vi "FunctionGenerator.vi"() -> ()   [LabVIEW 2017]
uses:
  waveformctrlFG.ctl
  FunctionGeneratorControls.ctl
  <vilib>/DAQmx/write.llb/DAQmx Write (Analog 1D DBL 1Chan NSamp).vi
  <vilib>/DAQmx/create/channels.llb/DAQmx Create Channel (AO-Voltage-Basic).vi
  <vilib>/DAQmx/configure/timing.llb/DAQmx Timing (Sample Clock).vi
  <vilib>/DAQmx/miscellaneous.llb/DAQmx Fill In Error Info.vi
  <resource>/objmgr/daqmx.rc
panel:
  in  "physical channels":tag="Dev8/ao0"
  in  "Frequency":dbl=1000.0 min=1.0 max=100000.0 step=1.0
  in  "Duty Cycle":dbl(knob)=0.5 min=0.1 max=0.99 step=0.1 scale=0.1..0.99
  in  "DC Offset":dbl(knob) min=-10.0 max=10.0 step=1.0 scale=-10.0..10.0
  in  "Amplitude":dbl(knob)=9.99 min=1.0 max=9.99 scale=1.0..10.0
  in  "Waveform":T1 items=["Sine", "Triangle", "Sawtooth", "Square", "TTL"]
  in  "stop":bool
  out "Waveform Graph":dbl[](graph)=[0.0, 0.07846046987822623, 0.15691609994508854, 0.23536205068776545, 0.31379348319050165, 0.39220555943309543, 0.4705934425893302, 0.5489522973253331, 0.6272772900978406, 0.7055635894523551, 0.783806366321171, 0.8620007943212546, 0.9401420500519582, 1.0182253133925498, 1.0962457677995423, 1.1741986006037983, 1.2520790033073996, 1.329882171880258, 1.4076033070564509, 1.4852376146302608, 1.5627803057519065, 1.6402265972229408, 1.7175717117913014, 1.7948108784459935, 1.8719393327113891, 1.9489523169411216, 2.02584508061156, 2.102612880614844, 2.1792509815514602, 2.2557546560223463, 2.332119184920495, 2.4083398577220563, 2.4844119727768996, 2.5603308375986367, 2.6360917691540755, 2.711690094152092, 2.7871211493319006, 2.8623802817507054, 2.937462849070717, 3.0123642198455123, 3.0870797738057245, 3.1616049021440453, 3.2359350077995126, 3.3100655057410844, 3.3839918232504616, 3.4577094002041555, 3.5312136893547788, 3.6045001566115418, 3.677564281319933, 3.750401556540578, 3.8230074893272477, 3.8953776010040007, 3.9675074274414586, 4.0393925193321625, 4.111028442465037, 4.182410777998907, 4.253535122735077, 4.324397089388936, 4.394992306860592, 4.4653164205045, 4.535365092398073, 4.60513400160927, 4.6746188444631285, 4.74381533480724, 4.812719204276136, 4.88132620255458, 4.949632097639752, 5.017632676102291, 5.085323743346209, 5.152701123867625, 5.219760661512328, 5.286498219732165, 5.352909681840177, 5.418990951264557, 5.484737951801336, 5.550146627865826, 5.615212944742785, 5.679932888835297, 5.744302467912353, 5.808317711355108, 5.871974670401807, 5.935269418391366, 5.9981980510055815, 6.060756686509977, 6.122941465993235, 6.1847485536052424, 6.246174136793695, 6.307214426539284, 6.367865657589411, 6.428124088690452, 6.487986002818536, 6.547447707408821, 6.606505534583282, 6.665155841376952, 6.723395009962635, 6.781219447874088, 6.8386255882276, 6.895609889942028, 6.952168837957221, 7.008298943450849, 7.06399674405361, 7.119258804062802, 7.174081714654257, 7.2284620940926105, 7.2823965879399015, 7.335881869262499, 7.388914638836311, 7.441491625350304, 7.493609585608292, 7.545265304728985, 7.596455596344311, 7.64717730279595, 7.697427295330135, 7.7472024742906225, 7.796499769309913, 7.845316139498642, 7.893648573633147, 7.9414940903412266, 7.988849738286035, 8.035712596348144, 8.082079773805726, 8.127948410512863, 8.173315677075985, 8.21817877502839, 8.262534937002872, 8.306381426902426, 8.34971554006902, 8.39253460345043, 8.43483597576513, 8.476617047665222, 8.51787524189738, 8.558608013461848, 8.598812849769397, 8.63848727079635, 8.67762882923753, 8.716235110657243, 8.7543037336382, 8.791832349928407, 8.828818644586049, 8.86526033612224, 8.901155176641794, 8.936500951981872, 8.97129548184855, 9.005536619951334, 9.039222254135536, 9.072350306512561, 9.104918733588098, 9.13692552638815, 9.168368710582971, 9.199246346608852, 9.229556529787756, 9.259297390444807, 9.288467094023632, 9.317063841199511, 9.345085867990374, 9.372531445865617, 9.399398881852713, 9.425686518641655, 9.451392734687177, 9.47651594430879, 9.501054597788585, 9.525007181466822, 9.548372217835318, 9.571148265628569, 9.593333919912661, 9.614927812171937, 9.635928610393403, 9.656335019148905, 9.676145779675025, 9.69535966995074, 9.71397550477279, 9.731992135828795, 9.749408451768087, 9.76622337827026, 9.78243587811144, 9.798044951228272, 9.8130496347796, 9.827449003205864, 9.841242168286191, 9.85442827919319, 9.867006522545427, 9.878976122457601, 9.89033634058841, 9.901086476186089, 9.911225866131634, 9.920753884979714, 9.929669944997245, 9.937973496199648, 9.945664026384769, 9.952741061164483, 9.959204163993949, 9.96505293619854, 9.970287016998434, 9.974906083530874, 9.97890985087008, 9.982298072044822, 9.985070538053659, 9.987227077877826, 9.988767558491789, 9.98969188487145, 9.99, 9.98969188487145, 9.988767558491789, 9.987227077877826, 9.985070538053659, 9.982298072044822, 9.97890985087008, 9.974906083530874, 9.970287016998434, 9.965052936198537, 9.959204163993949, 9.952741061164483, 9.945664026384769, 9.937973496199648, 9.929669944997245, 9.920753884979714, 9.911225866131634, 9.901086476186087, 9.89033634058841, 9.878976122457601, 9.867006522545426, 9.85442827919319, 9.841242168286191, 9.827449003205864, 9.813049634779599, 9.798044951228272, 9.78243587811144, 9.76622337827026, 9.749408451768087, 9.731992135828795, 9.713975504772788, 9.69535966995074, 9.676145779675025, 9.656335019148903, 9.635928610393403, 9.614927812171937, 9.593333919912661, 9.571148265628569, 9.548372217835318, 9.525007181466822, 9.501054597788585, 9.47651594430879, 9.451392734687177, 9.425686518641655, 9.399398881852713, 9.372531445865615, 9.345085867990374, 9.317063841199511, 9.288467094023632, 9.259297390444805, 9.229556529787756, 9.199246346608852, 9.168368710582971, 9.136925526388149, 9.104918733588098, 9.072350306512561, 9.039222254135534, 9.005536619951334, 8.97129548184855, 8.936500951981872, 8.901155176641796, 8.865260336122239, 8.828818644586045, 8.791832349928407, 8.754303733638196, 8.716235110657243, 8.67762882923753, 8.63848727079635, 8.598812849769397, 8.558608013461846, 8.517875241897382, 8.47661704766522, 8.43483597576513, 8.392534603450429, 8.349715540069019, 8.306381426902426, 8.262534937002872, 8.21817877502839, 8.173315677075983, 8.127948410512863, 8.082079773805726, 8.035712596348143, 7.988849738286033, 7.941494090341224, 7.893648573633146, 7.8453161394986415, 7.796499769309913, 7.7472024742906225, 7.697427295330135, 7.64717730279595, 7.596455596344309, 7.545265304728983, 7.493609585608289, 7.441491625350303, 7.38891463883631, 7.335881869262498, 7.282396587939901, 7.228462094092609, 7.174081714654257, 7.119258804062802, 7.06399674405361, 7.008298943450846, 6.952168837957219, 6.895609889942025, 6.838625588227599, 6.781219447874087, 6.723395009962635, 6.665155841376951, 6.606505534583282, 6.547447707408821, 6.487986002818536, 6.428124088690449, 6.367865657589409, 6.307214426539281, 6.246174136793694, 6.184748553605241, 6.122941465993234, 6.0607566865099765, 5.9981980510055815, 5.935269418391366, 5.871974670401808, 5.808317711355105, 5.744302467912351, 5.679932888835295, 5.615212944742783, 5.550146627865826, 5.4847379518013355, 5.418990951264556, 5.352909681840177, 5.286498219732165, 5.219760661512327, 5.1527011238676215, 5.0853237433462075, 5.01763267610229, 4.94963209763975, 4.881326202554579, 4.812719204276135, 4.74381533480724, 4.6746188444631285, 4.60513400160927, 4.535365092398069, 4.4653164205044975, 4.3949923068605905, 4.324397089388934, 4.253535122735074, 4.182410777998905, 4.111028442465036, 4.0393925193321625, 3.9675074274414586, 3.8953776010040015, 3.8230074893272437, 3.750401556540575, 3.6775642813199307, 3.60450015661154, 3.5312136893547774, 3.4577094002041537, 3.38399182325046, 3.310065505741084, 3.235935007799513, 3.161604902144046, 3.087079773805722, 3.012364219845509, 2.937462849070714, 2.862380281750703, 2.787121149331899, 2.711690094152091, 2.6360917691540746, 2.5603308375986362, 2.4844119727768996, 2.408339857722057, 2.332119184920492, 2.255754656022343, 2.1792509815514576, 2.1026128806148416, 2.025845080611558, 1.9489523169411205, 1.8719393327113885, 1.7948108784459935, 1.7175717117913016, 1.6402265972229415, 1.5627803057519032, 1.485237614630258, 1.4076033070564484, 1.3298821718802563, 1.2520790033073979, 1.1741986006037972, 1.0962457677995416, 1.0182253133925498, 0.9401420500519584, 0.8620007943212509, 0.7838063663211678, 0.7055635894523523, 0.6272772900978383, 0.5489522973253311, 0.4705934425893287, 0.3922055594330944, 0.3137934831905011, 0.23536205068776533, 0.1569160999450889, 0.07846046987822257, -3.21302905405392e-15, -0.07846046987822898, -0.15691609994509087, -0.2353620506877673, -0.3137934831905031, -0.3922055594330964, -0.4705934425893307, -0.5489522973253331, -0.6272772900978404, -0.7055635894523589, -0.7838063663211742, -0.8620007943212573, -0.9401420500519604, -1.0182253133925516, -1.0962457677995436, -1.174198600603799, -1.2520790033073999, -1.329882171880258, -1.4076033070564502, -1.4852376146302644, -1.5627803057519094, -1.6402265972229435, -1.7175717117913036, -1.7948108784459953, -1.8719393327113905, -1.9489523169411223, -2.02584508061156, -2.102612880614844, -2.17925098155146, -2.2557546560223494, -2.332119184920498, -2.408339857722059, -2.484411972776902, -2.5603308375986384, -2.636091769154077, -2.7116900941520923, -2.7871211493319006, -2.8623802817507054, -2.937462849070716, -3.012364219845515, -3.087079773805728, -3.1616049021440475, -3.235935007799515, -3.310065505741086, -3.383991823250462, -3.457709400204156, -3.5312136893547788, -3.6045001566115418, -3.6775642813199365, -3.7504015565405813, -3.82300748932725, -3.8953776010040038, -3.9675074274414603, -4.039392519332164, -4.111028442465038, -4.182410777998907, -4.253535122735076, -4.324397089388935, -4.394992306860596, -4.465316420504503, -4.5353650923980755, -4.605134001609271, -4.67461884446313, -4.743815334807242, -4.812719204276137, -4.881326202554581, -4.949632097639752, -5.017632676102291, -5.085323743346213, -5.152701123867627, -5.219760661512332, -5.286498219732166, -5.352909681840178, -5.418990951264558, -5.484737951801336, -5.550146627865827, -5.615212944742785, -5.679932888835297, -5.744302467912356, -5.8083177113551105, -5.871974670401809, -5.935269418391367, -5.998198051005583, -6.060756686509978, -6.122941465993236, -6.1847485536052424, -6.246174136793695, -6.307214426539284, -6.367865657589413, -6.4281240886904545, -6.487986002818537, -6.547447707408824, -6.606505534583284, -6.665155841376952, -6.723395009962637, -6.781219447874088, -6.8386255882276, -6.895609889942028, -6.952168837957222, -7.008298943450851, -7.063996744053611, -7.119258804062804, -7.174081714654258, -7.2284620940926105, -7.2823965879399015, -7.335881869262499, -7.388914638836311, -7.441491625350304, -7.493609585608294, -7.5452653047289875, -7.5964555963443114, -7.647177302795949, -7.697427295330136, -7.747202474290626, -7.796499769309915, -7.845316139498646, -7.893648573633147, -7.941494090341228, -7.988849738286034, -8.035712596348146, -8.082079773805724, -8.127948410512865, -8.173315677075987, -8.21817877502839, -8.262534937002876, -8.306381426902426, -8.349715540069022, -8.39253460345043, -8.434835975765132, -8.47661704766522, -8.517875241897384, -8.558608013461845, -8.598812849769399, -8.638487270796352, -8.67762882923753, -8.716235110657246, -8.754303733638197, -8.791832349928411, -8.828818644586047, -8.86526033612224, -8.901155176641794, -8.936500951981872, -8.971295481848554, -9.005536619951336, -9.039222254135538, -9.072350306512563, -9.1049187335881, -9.136925526388149, -9.168368710582973, -9.199246346608852, -9.229556529787756, -9.259297390444805, -9.288467094023632, -9.317063841199513, -9.345085867990376, -9.372531445865619, -9.399398881852713, -9.425686518641655, -9.451392734687177, -9.476515944308792, -9.501054597788585, -9.525007181466822, -9.54837221783532, -9.571148265628569, -9.593333919912663, -9.614927812171937, -9.635928610393405, -9.656335019148903, -9.676145779675025, -9.69535966995074, -9.71397550477279, -9.731992135828794, -9.749408451768087, -9.76622337827026, -9.78243587811144, -9.798044951228274, -9.8130496347796, -9.827449003205864, -9.841242168286191, -9.85442827919319, -9.867006522545426, -9.878976122457601, -9.89033634058841, -9.901086476186089, -9.911225866131634, -9.920753884979714, -9.929669944997245, -9.937973496199648, -9.945664026384769, -9.952741061164483, -9.959204163993949, -9.96505293619854, -9.970287016998434, -9.974906083530874, -9.97890985087008, -9.982298072044822, -9.985070538053659, -9.987227077877826, -9.988767558491789, -9.98969188487145, -9.99, -9.98969188487145, -9.988767558491789, -9.987227077877826, -9.985070538053657, -9.982298072044822, -9.97890985087008, -9.974906083530874, -9.970287016998434, -9.96505293619854, -9.959204163993949, -9.952741061164483, -9.945664026384769, -9.937973496199646, -9.929669944997245, -9.920753884979714, -9.911225866131634, -9.901086476186087, -9.89033634058841, -9.878976122457601, -9.867006522545427, -9.85442827919319, -9.841242168286191, -9.827449003205864, -9.813049634779599, -9.798044951228272, -9.782435878111439, -9.76622337827026, -9.749408451768087, -9.731992135828795, -9.713975504772788, -9.695359669950738, -9.676145779675025, -9.656335019148903, -9.635928610393403, -9.614927812171935, -9.593333919912661, -9.571148265628569, -9.548372217835318, -9.525007181466822, -9.501054597788585, -9.47651594430879, -9.451392734687175, -9.425686518641653, -9.399398881852711, -9.372531445865617, -9.345085867990374, -9.317063841199511, -9.28846709402363, -9.259297390444807, -9.229556529787754, -9.199246346608849, -9.168368710582971, -9.136925526388149, -9.104918733588098, -9.072350306512561, -9.039222254135536, -9.005536619951334, -8.97129548184855, -8.93650095198187, -8.901155176641792, -8.865260336122239, -8.828818644586045, -8.791832349928407, -8.754303733638196, -8.716235110657243, -8.677628829237529, -8.63848727079635, -8.598812849769395, -8.558608013461848, -8.51787524189738, -8.476617047665219, -8.43483597576513, -8.392534603450427, -8.349715540069019, -8.306381426902425, -8.262534937002872, -8.218178775028388, -8.173315677075985, -8.127948410512861, -8.08207977380572, -8.035712596348143, -7.988849738286031, -7.941494090341226, -7.893648573633144, -7.845316139498642, -7.796499769309912, -7.7472024742906225, -7.697427295330132, -7.647177302795952, -7.596455596344308, -7.54526530472898, -7.49360958560829, -7.4414916253503005, -7.388914638836311, -7.335881869262495, -7.2823965879399015, -7.228462094092607, -7.174081714654258, -7.119258804062801, -7.063996744053605, -7.008298943450847, -6.952168837957216, -6.895609889942026, -6.838625588227596, -6.781219447874087, -6.723395009962633, -6.665155841376952, -6.606505534583279, -6.547447707408816, -6.487986002818532, -6.428124088690447, -6.36786565758941, -6.3072144265392796, -6.246174136793694, -6.184748553605238, -6.122941465993235, -6.060756686509974, -5.998198051005582, -5.935269418391362, -5.871974670401801, -5.808317711355106, -5.744302467912348, -5.679932888835297, -5.6152129447427805, -5.550146627865826, -5.484737951801332, -5.418990951264557, -5.352909681840173, -5.286498219732159, -5.2197606615123275, -5.152701123867619, -5.085323743346208, -5.017632676102287, -4.949632097639751, -4.881326202554576, -4.812719204276136, -4.743815334807238, -4.674618844463129, -4.605134001609267, -4.535365092398067, -4.465316420504498, -4.394992306860587, -4.324397089388935, -4.253535122735071, -4.182410777998906, -4.111028442465034, -4.039392519332163, -3.967507427441456, -3.895377601003995, -3.823007489327245, -3.7504015565405724, -3.677564281319932, -3.6045001566115364, -3.5312136893547783, -3.457709400204151, -3.3839918232504616, -3.3100655057410813, -3.2359350077995144, -3.1616049021440427, -3.0870797738057183, -3.01236421984551, -2.937462849070711, -2.8623802817507045, -2.7871211493318957, -2.711690094152092, -2.6360917691540715, -2.560330837598637, -2.4844119727768965, -2.4083398577220496, -2.3321191849204927, -2.25575465602234, -2.179250981551459, -2.1026128806148385, -2.0258450806115595, -1.9489523169411174, -1.8719393327113896, -1.7948108784459902, -1.7175717117912943, -1.6402265972229384, -1.5627803057519, -1.485237614630259, -1.4076033070564453, -1.3298821718802574, -1.2520790033073947, -1.1741986006037983, -1.0962457677995385, -1.018225313392551, -0.9401420500519552, -0.8620007943212477, -0.7838063663211691, -0.7055635894523491, -0.6272772900978395, -0.5489522973253279, -0.47059344258932995, -0.3922055594330912, -0.3137934831905023, -0.23536205068776211, -0.15691609994508124, -0.07846046987822379]
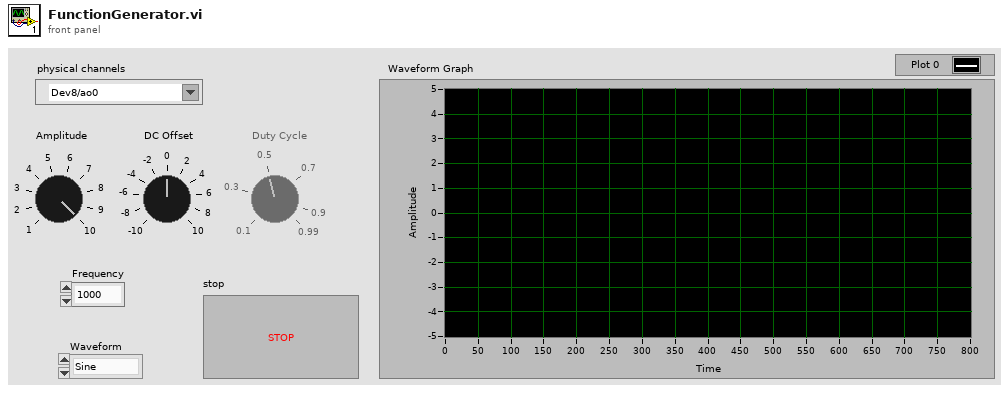
[diagram p1: front panel]
types:
  T1 = typedef "waveformctrlFG.ctl" = u16
  T2 = enum8{"Enabled", "Disabled", "Disabled and Grayed Out"}
  T3 = typedef "FunctionGeneratorControls.ctl" = enum16{"Intialize", "Wait for UI", "Output", "Stop"}
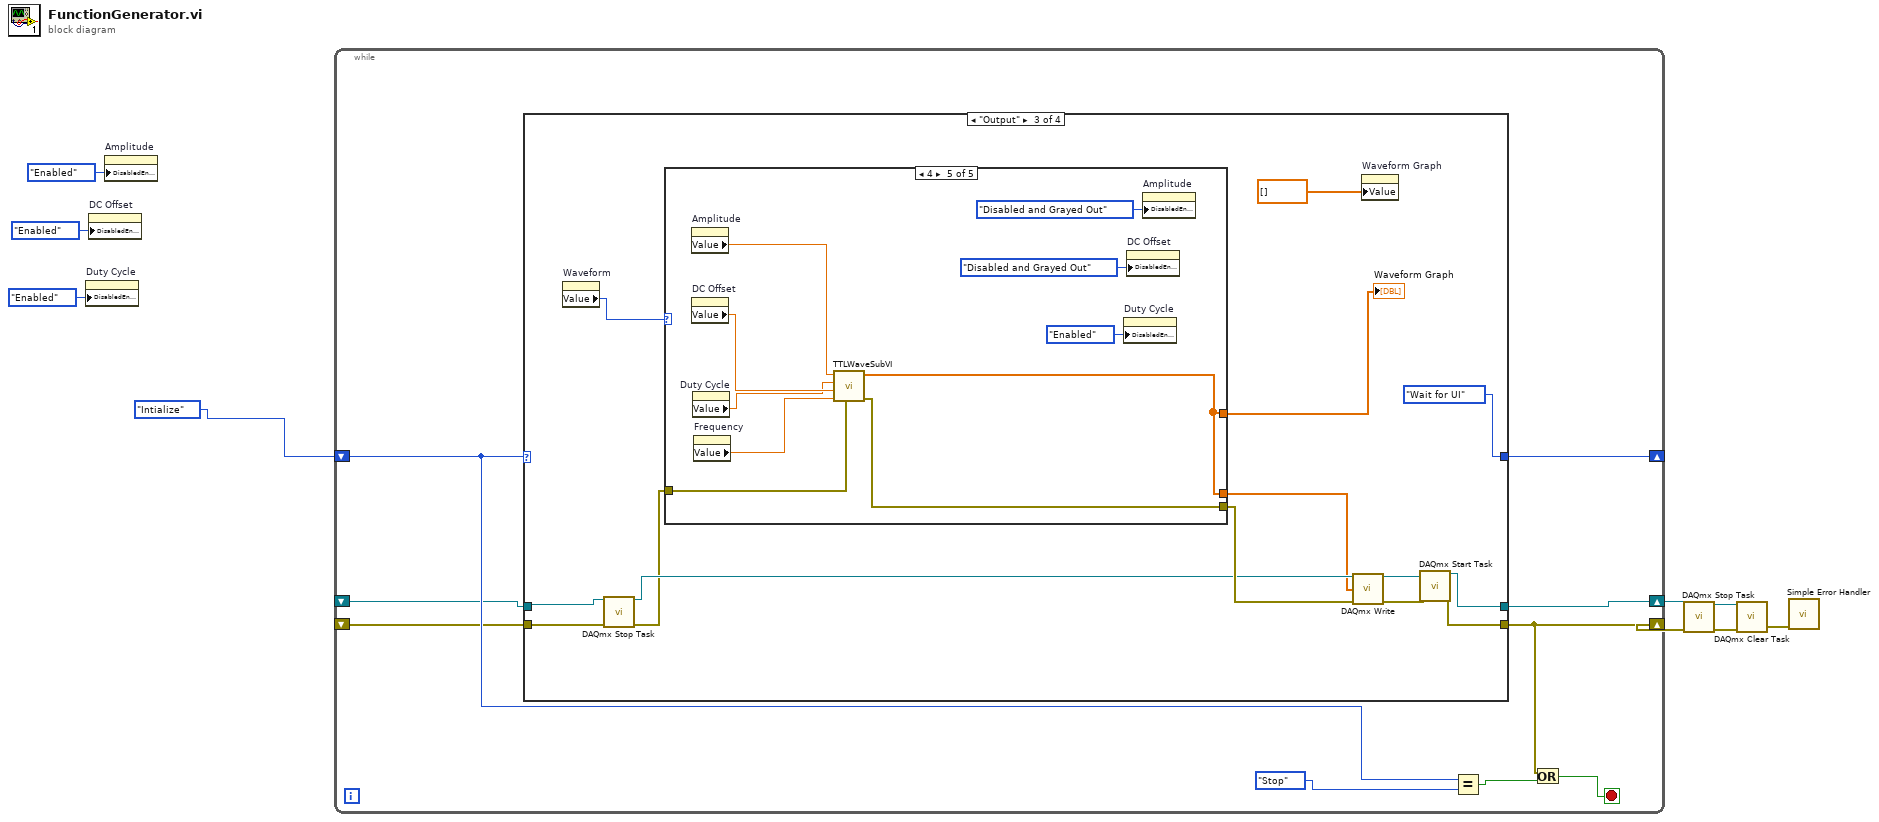
[diagram p0: block diagram]
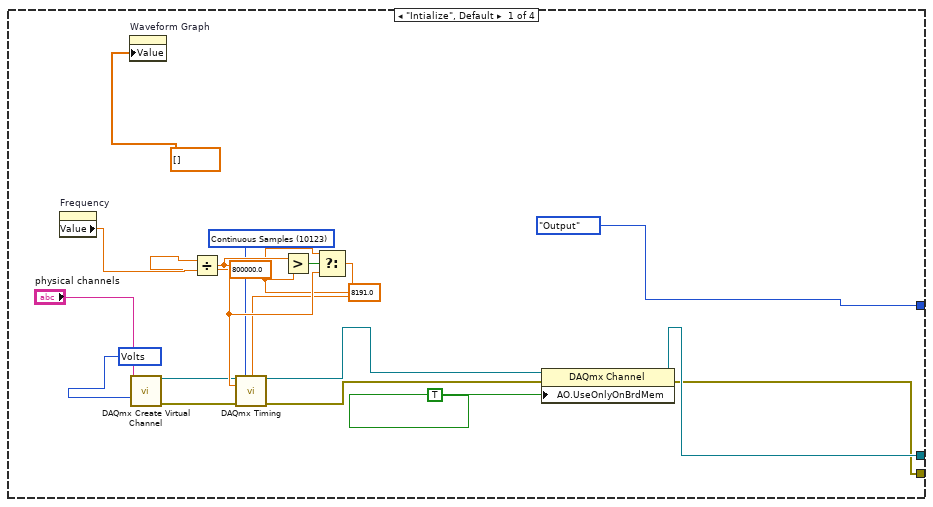
[diagram p2: hidden frame]
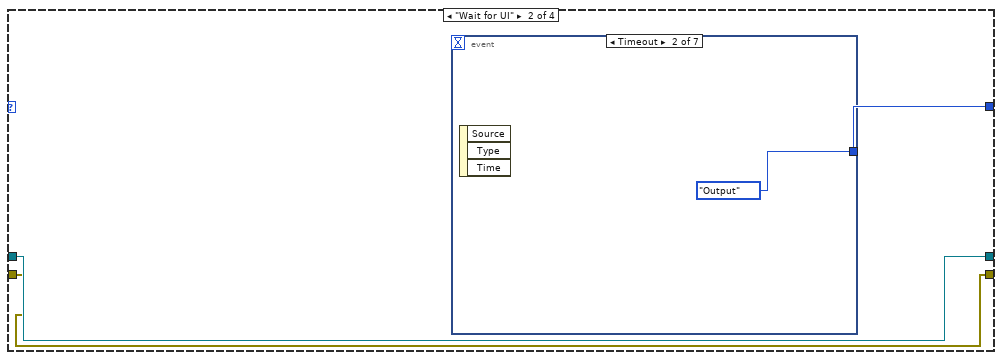
[diagram p3: hidden frame]
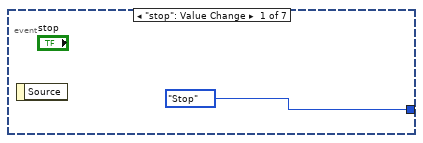
[diagram p4: hidden frame]
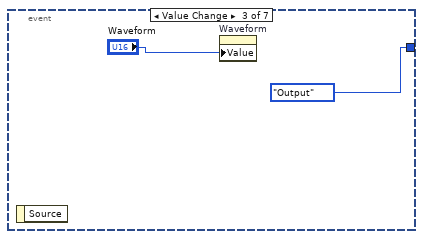
[diagram p5: hidden frame]
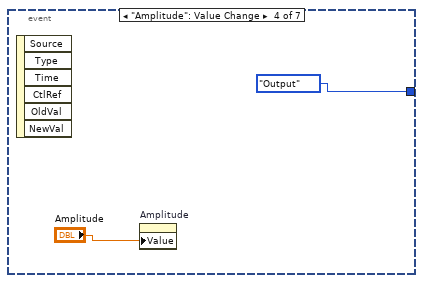
[diagram p6: hidden frame]
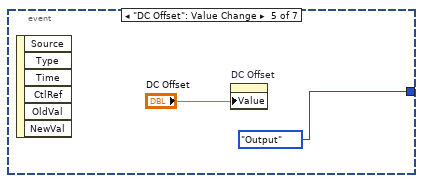
[diagram p7: hidden frame]
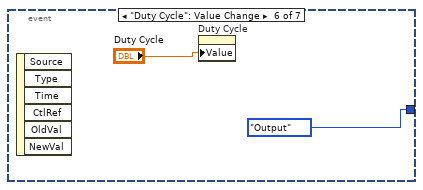
[diagram p8: hidden frame]
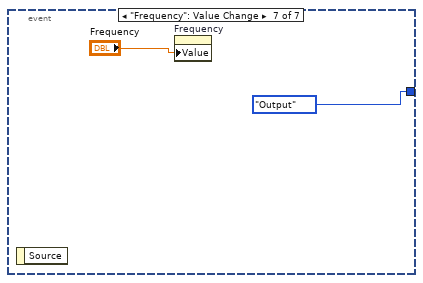
[diagram p9: hidden frame]
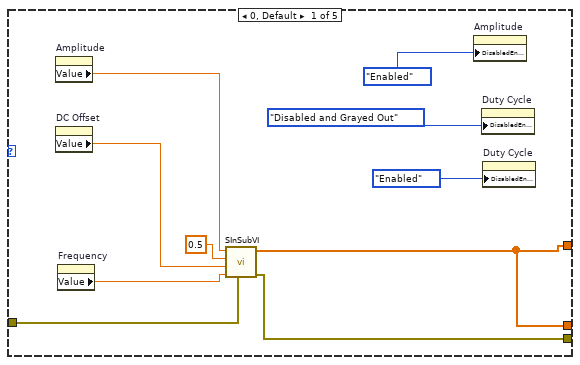
[diagram p10: hidden frame]
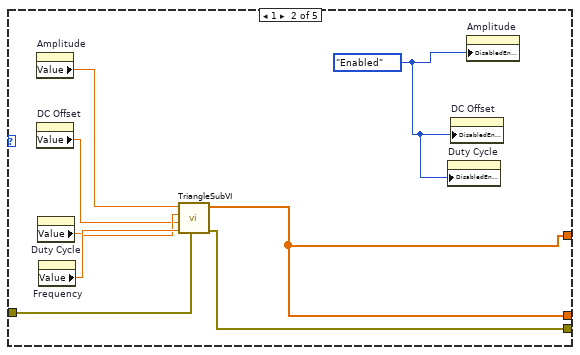
[diagram p11: hidden frame]
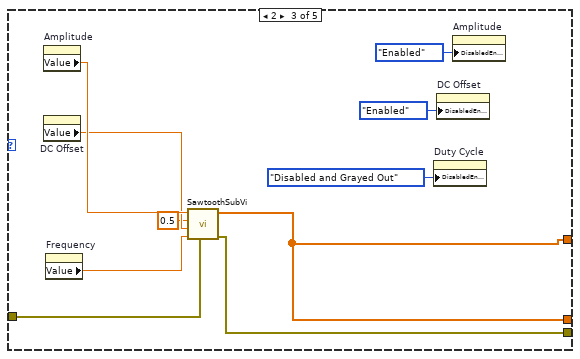
[diagram p12: hidden frame]
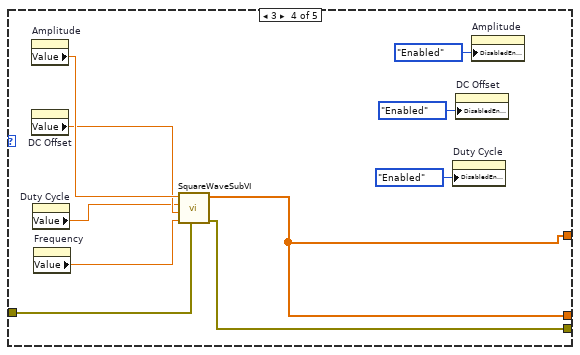
[diagram p13: hidden frame]
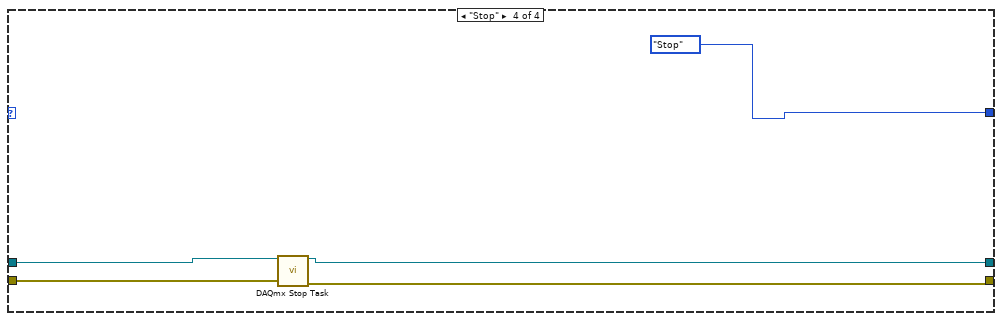
[diagram p14: hidden frame]
diagram:
  n1 = property on="Duty Cycle" class="Knob (strict)"("DisabledEnum"=T2."Enabled" ("Disabled")) -> ()  [unwired: 2 in, 2 out]
  n2 = property on="DC Offset" class="Knob (strict)"("DisabledEnum"=T2."Enabled" ("Disabled")) -> ()  [unwired: 2 in, 2 out]
  n3 = property on="Amplitude" class="Knob (strict)"("DisabledEnum"=T2."Enabled" ("Disabled")) -> ()  [unwired: 2 in, 2 out]
  n4 = while {
    shift-right: [w18] -> _
    shift-left: FunctionGeneratorControls."Intialize" -> [w16]
    shift-right: [w15] -> w9
    shift-left: _ -> [w11]
    shift-right: [w12] -> w8
    shift-left: _ -> [w10]
    stop <- w13 stop-if-true
    n5 = case shown="\"Output\"" w16 {
      tunnel: [FunctionGeneratorControls."Output" w39 FunctionGeneratorControls."Wait for UI" FunctionGeneratorControls."Stop"] -> w18
      tunnel: w11 -> [_ w38 w59 w118]
      tunnel: w10 -> [_ w37 w58 w117]
      tunnel: [w21 w38 w55 w116] -> w15
      tunnel: [w20 w37 w54 w115] -> w12
      frame "Intialize", Default {
        w26 = 8191.0 ("y")
        w23 = 10123 items=["Finite Samples"=10178, "Continuous Samples"=10123, "Hardware Timed Single Point"=12522] ("sample mode")
        w22 = 10348 items=["Volts"=10348, "From Custom Scale"=10065] ("units")
        n6 = property on="Frequency" class="DigNum (strict)"() -> ("Value"=w35:dbl)  [unwired: 2 in, 2 out]
        n7 = property on="Waveform Graph" class="WFGraph (strict)"("Value"=dbl[] [] ("Waveform Graph")) -> ()  [unwired: 2 in, 2 out]
        n8 = call-poly <vilib>:"DAQmx Create Virtual Channel.vi"("physical channels"="physical channels", "units"=w22) -> ("task out"=w27:refnum<k21>, "error out"=w28:errorcluster)  [unwired: 12 in]
        n9 = Divide(x=800000.0, y=w35) -> (x/y=w32:dbl)
        n10 = Greater?(x=w32, y=w26) -> (0:w30:bool)
        n11 = Select(t=w26, s=w30, f=w32) -> (s? t:f=w31:dbl)
        n12 = call-poly <vilib>:"DAQmx Timing.vi"("task/channels in"=w27, "sample mode"=w23, "samples per channel"=w31, "rate"=w32, "error in"=w28) -> ("task out"=w33:refnum<k21>, "error out"=w29:errorcluster)  [unwired: 9 in]
        n13 = property class="DAQmx Channel"(reference=w33, error in=w29, "AO.UseOnlyOnBrdMem"=TRUE) -> (reference out=w21:refnum<k21>, error out=w20:errorcluster)
      }
      frame "Wait for UI" {
        n14 = event shown="[1] Timeout" {
          selector: _ -> [_ _ _ _ _ _ _]
          dyn-events: _ -> [_ _ _ _ _ _ _]
          timeout: _ -> [_ _ _ _ _ _ _]
          tunnel: [FunctionGeneratorControls."Stop" FunctionGeneratorControls."Output" FunctionGeneratorControls."Output" FunctionGeneratorControls."Output" FunctionGeneratorControls."Output" FunctionGeneratorControls."Output" FunctionGeneratorControls."Output"] -> w39
          event "stop": Value Change {
            n15 = event-data() -> ()  [unwired: 1 in, 1 out]
          }
          event Timeout {
            n16 = event-data() -> ()  [unwired: 1 in, 3 out]
          }
          event Value Change {
            n17 = event-data() -> ()  [unwired: 1 in, 1 out]
            n18 = property on="Waveform" class="Ring (strict)"("Value"="Waveform") -> ()  [unwired: 2 in, 2 out]
          }
          event "Amplitude": Value Change {
            n19 = event-data() -> ()  [unwired: 1 in, 6 out]
            n20 = property on="Amplitude" class="Knob (strict)"("Value"="Amplitude") -> ()  [unwired: 2 in, 2 out]
          }
          event "DC Offset": Value Change {
            n21 = event-data() -> ()  [unwired: 1 in, 6 out]
            n22 = property on="DC Offset" class="Knob (strict)"("Value"="DC Offset") -> ()  [unwired: 2 in, 2 out]
          }
          event "Duty Cycle": Value Change {
            n23 = event-data() -> ()  [unwired: 1 in, 6 out]
            n24 = property on="Duty Cycle" class="Knob (strict)"("Value"="Duty Cycle") -> ()  [unwired: 2 in, 2 out]
          }
          event "Frequency": Value Change {
            n25 = event-data() -> ()  [unwired: 1 in, 1 out]
            n26 = property on="Frequency" class="DigNum (strict)"("Value"="Frequency") -> ()  [unwired: 2 in, 2 out]
          }
        }
      }
      frame "Output" {
        n27 = property on="Waveform" class="Ring (strict)"() -> ("Value"=w62:T1)  [unwired: 2 in, 2 out]
        n28 = call <vilib>:"DAQmx Stop Task.vi"("task/channels in"=w59, "error in"=w58) -> ("task out"=w57:refnum<k21>, "error out"=w56:errorcluster)  [unwired: 12 in]
        n29 = case shown="4" w62 {
          tunnel: w56 -> [w75 w83 w93 w103 w113]
          tunnel: [w74 w82 w92 w102 w112] -> w61
          tunnel: [w70 w77 w88 w97 w107] -> w53
          tunnel: [w70 w77 w88 w97 w107] -> w52
          frame 0, Default {
            n30 = property on="Amplitude" class="Knob (strict)"() -> ("Value"=w71:dbl)  [unwired: 2 in, 2 out]
            n31 = property on="DC Offset" class="Knob (strict)"() -> ("Value"=w72:dbl)  [unwired: 2 in, 2 out]
            n32 = property on="Frequency" class="DigNum (strict)"() -> ("Value"=w73:dbl)  [unwired: 2 in, 2 out]
            n33 = call "SInSubVI.vi"("Error In"=w75, "Frequency"=w73, "DC Offset"=w72, "Duty Cycle"=0.5, "Amplitude"=w71) -> ("Error Out"=w74:errorcluster, "Array"=w70:dbl[])  [unwired: 5 in]
            n34 = property on="Amplitude" class="Knob (strict)"("DisabledEnum"=T2."Enabled" ("Disabled")) -> ()  [unwired: 2 in, 2 out]
            n35 = property on="Duty Cycle" class="Knob (strict)"("DisabledEnum"=T2."Disabled and Grayed Out" ("Disabled")) -> ()  [unwired: 2 in, 2 out]
            n36 = property on="Duty Cycle" class="Knob (strict)"("DisabledEnum"=T2."Enabled" ("Disabled")) -> ()  [unwired: 2 in, 2 out]
          }
          frame 1 {
            w76 = T2."Enabled" ("Disabled")
            n37 = property on="Amplitude" class="Knob (strict)"() -> ("Value"=w78:dbl)  [unwired: 2 in, 2 out]
            n38 = property on="DC Offset" class="Knob (strict)"() -> ("Value"=w79:dbl)  [unwired: 2 in, 2 out]
            n39 = property on="Duty Cycle" class="Knob (strict)"() -> ("Value"=w80:dbl)  [unwired: 2 in, 2 out]
            n40 = property on="Frequency" class="DigNum (strict)"() -> ("Value"=w81:dbl)  [unwired: 2 in, 2 out]
            n41 = call "TriangleSubVI.vi"("Error In"=w83, "Frequency"=w81, "DC Offset"=w79, "Duty Cycle"=w80, "Amplitude"=w78) -> ("Error Out"=w82:errorcluster, "Array"=w77:dbl[])  [unwired: 5 in]
            n42 = property on="Duty Cycle" class="Knob (strict)"("DisabledEnum"=w76) -> ()  [unwired: 2 in, 2 out]
            n43 = property on="DC Offset" class="Knob (strict)"("DisabledEnum"=w76) -> ()  [unwired: 2 in, 2 out]
            n44 = property on="Amplitude" class="Knob (strict)"("DisabledEnum"=w76) -> ()  [unwired: 2 in, 2 out]
          }
          frame 2 {
            n45 = property on="Amplitude" class="Knob (strict)"() -> ("Value"=w91:dbl)  [unwired: 2 in, 2 out]
            n46 = property on="DC Offset" class="Knob (strict)"() -> ("Value"=w90:dbl)  [unwired: 2 in, 2 out]
            n47 = property on="Frequency" class="DigNum (strict)"() -> ("Value"=w89:dbl)  [unwired: 2 in, 2 out]
            n48 = call "SawtoothSubVi.vi"("Error In"=w93, "Frequency"=w89, "DC Offset"=w90, "Duty Cycle"=0.5, "Amp"=w91) -> ("Error Out"=w92:errorcluster, "Array"=w88:dbl[])  [unwired: 5 in]
            n49 = property on="Duty Cycle" class="Knob (strict)"("DisabledEnum"=T2."Disabled and Grayed Out" ("Disabled")) -> ()  [unwired: 2 in, 2 out]
            n50 = property on="DC Offset" class="Knob (strict)"("DisabledEnum"=T2."Enabled" ("Disabled")) -> ()  [unwired: 2 in, 2 out]
            n51 = property on="Amplitude" class="Knob (strict)"("DisabledEnum"=T2."Enabled" ("Disabled")) -> ()  [unwired: 2 in, 2 out]
          }
          frame 3 {
            n52 = property on="Amplitude" class="Knob (strict)"() -> ("Value"=w101:dbl)  [unwired: 2 in, 2 out]
            n53 = property on="DC Offset" class="Knob (strict)"() -> ("Value"=w100:dbl)  [unwired: 2 in, 2 out]
            n54 = property on="Duty Cycle" class="Knob (strict)"() -> ("Value"=w99:dbl)  [unwired: 2 in, 2 out]
            n55 = property on="Frequency" class="DigNum (strict)"() -> ("Value"=w98:dbl)  [unwired: 2 in, 2 out]
            n56 = call "SquareWaveSubVI.vi"("Error In"=w103, "Frequency"=w98, "DC Off"=w100, "Duty Cycle"=w99, "Amplitude"=w101) -> ("Error Out"=w102:errorcluster, "Array"=w97:dbl[])  [unwired: 5 in]
            n57 = property on="Duty Cycle" class="Knob (strict)"("DisabledEnum"=T2."Enabled" ("Disabled")) -> ()  [unwired: 2 in, 2 out]
            n58 = property on="DC Offset" class="Knob (strict)"("DisabledEnum"=T2."Enabled" ("Disabled")) -> ()  [unwired: 2 in, 2 out]
            n59 = property on="Amplitude" class="Knob (strict)"("DisabledEnum"=T2."Enabled" ("Disabled")) -> ()  [unwired: 2 in, 2 out]
          }
          frame 4 {
            n60 = property on="Amplitude" class="Knob (strict)"() -> ("Value"=w111:dbl)  [unwired: 2 in, 2 out]
            n61 = property on="DC Offset" class="Knob (strict)"() -> ("Value"=w110:dbl)  [unwired: 2 in, 2 out]
            n62 = property on="Duty Cycle" class="Knob (strict)"() -> ("Value"=w109:dbl)  [unwired: 2 in, 2 out]
            n63 = property on="Frequency" class="DigNum (strict)"() -> ("Value"=w108:dbl)  [unwired: 2 in, 2 out]
            n64 = call "TTLWaveSubVI.vi"("Error In"=w113, "Frequency"=w108, "DC Offset"=w110, "Duty Cycle"=w109, "Amplitude"=w111) -> ("Error Out"=w112:errorcluster, "Array"=w107:dbl[])  [unwired: 5 in]
            n65 = property on="Duty Cycle" class="Knob (strict)"("DisabledEnum"=T2."Enabled" ("Disabled")) -> ()  [unwired: 2 in, 2 out]
            n66 = property on="DC Offset" class="Knob (strict)"("DisabledEnum"=T2."Disabled and Grayed Out" ("Disabled")) -> ()  [unwired: 2 in, 2 out]
            n67 = property on="Amplitude" class="Knob (strict)"("DisabledEnum"=T2."Disabled and Grayed Out" ("Disabled")) -> ()  [unwired: 2 in, 2 out]
          }
        }
        "Waveform Graph" <- w52
        n68 = call-poly <vilib>:"DAQmx Write.vi"("task/channels in"=w57, "data"=w53, "error in"=w61) -> ("task out"=w65:refnum<k21>, "error out"=w64:errorcluster)  [unwired: 10 in, 1 out]
        n69 = property on="Waveform Graph" class="WFGraph (strict)"("Value"=dbl[] [] ("Waveform Graph")) -> ()  [unwired: 2 in, 2 out]
        n70 = call <vilib>:"DAQmx Start Task.vi"("task/channels in"=w65, "error in"=w64) -> ("task out"=w55:refnum<k21>, "error out"=w54:errorcluster)  [unwired: 12 in]
      }
      frame "Stop" {
        n71 = call <vilib>:"DAQmx Stop Task.vi"("task/channels in"=w118, "error in"=w117) -> ("task out"=w116:refnum<k21>, "error out"=w115:errorcluster)  [unwired: 12 in]
      }
    }
    n72 = Equal?(x=w16, y=FunctionGeneratorControls."Stop") -> (x = y?=w14:bool)
    n73 = Or(x=w12, y=w14) -> (x .or. y?=w13:bool)
  }
  n74 = call <vilib>:"DAQmx Stop Task.vi"("task/channels in"=w9, "error in"=w8) -> ("task out"=w7:refnum<k21>, "error out"=w6:errorcluster)  [unwired: 12 in]
  n75 = call <vilib>:"DAQmx Clear Task.vi"("task in"=w7, "error in"=w6) -> ("error out"=w5:errorcluster)  [unwired: 13 in]
  n76 = call <vilib>:"Simple Error Handler.vi"("error in (no error)"=w5) -> ()  [unwired: 4 in, 5 out]
